vi "FPGA_ReadAI.vi"(8 "error in (no error)":errorcluster, 9 "average?":bool, 10 "Channel":T1, 11 "AI Reference":T2) -> (0 "error out":errorcluster, 2 "Value":i32, 3 "AI Reference":T2)   [LabVIEW 2017]
uses:
  <vilib>/Rock Robotics/SystemInterfaces/AI/FPGA_AIDevRef.ctl
  <vilib>/Rock Robotics/SystemInterfaces/AI/FPGA_AIChannel.ctl
  <vilib>/Rock Robotics/SystemInterfaces/System/FPGA_SystemFPGA Ref Global.vi
  <vilib>/Utility/error.llb/Error Cluster From Error Code.vi
  <vilib>/rvi/errors/niLvFpgaAdjustHostInterfaceError.vi
  <vilib>/rvi/interface/nirviReadWriteControl/nirviReadWriteControl.xnode
  <vilib>/Rock Robotics/SystemInterfaces/System/FPGA_SystemFRC FPGA Ref.ctl
  <vilib>/rvi/interface/Simulation/niFpgaSimulationCallBeginRW.vi
  NiFpgaLv.dll
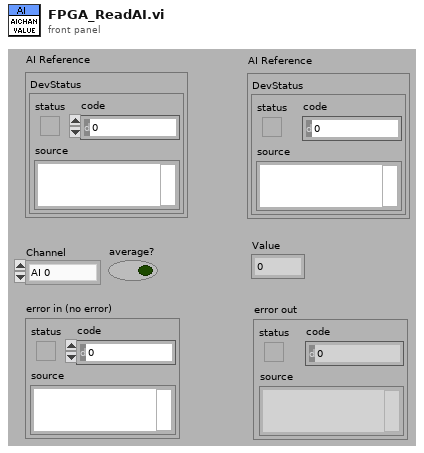
[diagram p1: front panel]
types:
  T1 = typedef "FPGA_AIChannel.ctl" = enum8{"AI 0", "AI 1", "AI 2", "AI 3", "AI MXP 0", "AI MXP 1", "AI MXP 2", "AI MXP 3", "Invalid"}
  T2 = typedef "FPGA_AIDevRef.ctl" = cluster{"DevStatus":errorcluster}
  T3 = typedef "FPGA_SystemFRC FPGA Ref.ctl" = refnum<k20>
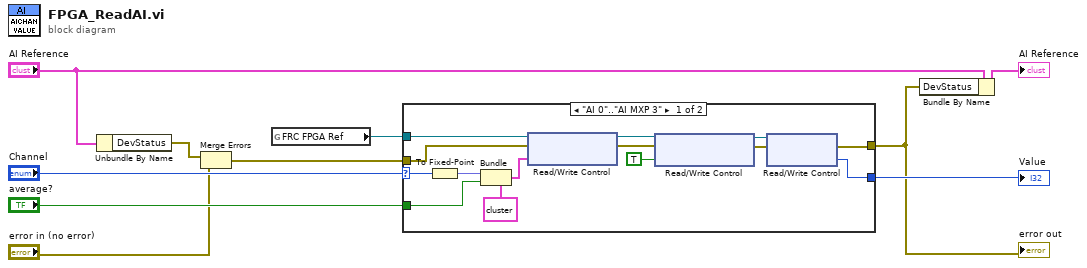
[diagram p0: block diagram]
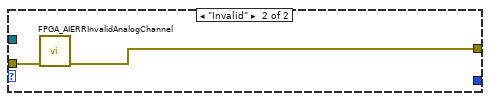
[diagram p2: hidden frame]
diagram:
  n1 = Unbundle By Name("AI Reference") -> ("DevStatus"=w5:errorcluster)
  n2 = Merge Errors(w5, "error in (no error)") -> (w4:errorcluster)
  n3 = global read "FPGA_SystemFPGA Ref Global.vi" "FRC FPGA Ref"() -> (w3:T3)
  n4 = case shown="\"AI 0\"..\"AI MXP 3\"" "Channel" {
    selector: "Channel" -> [w15 _]
    tunnel: w3 -> [w23 _]
    tunnel: w4 -> [w24 w26]
    tunnel: [w18 w25] -> w9
    tunnel: [w17 _] -> w10
    tunnel: "average?" -> [w11 _]
    frame "AI 0".."AI MXP 3" {
      n5 = To Fixed-Point(number=w15) -> (fixed-point=w13:fxp<+,3,3>)  [unwired: 1 out]
      n6 = Bundle(cluster=cluster{"Channel":fxp<+,3,3>, "Averaged":bool} {"Channel"=0.0, "Averaged"=FALSE} ("AI.ReadSelect"), "Channel"=w13, "Averaged"=w11) -> (w14:cluster{"Channel":fxp<+,3,3>, "Averaged":bool})
      n7 = xnode "Read/Write Control"("FPGA VI Reference In"=w23, "error in"=w24, "AI.ReadSelect"=w14) -> ("FPGA VI Reference Out"=w19:T3, "error out"=w20:errorcluster)
      n8 = xnode "Read/Write Control"("FPGA VI Reference In"=w19, "error in"=w20, "AI.LatchOutput"=TRUE) -> ("FPGA VI Reference Out"=w22:T3, "error out"=w21:errorcluster)
      n9 = xnode "Read/Write Control"("FPGA VI Reference In"=w22, "error in"=w21) -> ("error out"=w18:errorcluster, "AI.Output"=w17:i32)  [unwired: 1 out]
    }
    frame "Invalid" {
      n10 = call <vilib>:"FPGA_AIERRInvalidAnalogChannel.vi"("error in (no error)"=w26) -> ("error out"=w25:errorcluster)  [unwired: 10 in]
    }
  }
  "Value" <- w10
  "error out" <- w9
  n11 = Bundle By Name(cluster="AI Reference", "DevStatus"=w9) -> (→"AI Reference":T2)
